vi "Composite User Interface Launcher.vi"   [LabVIEW 2020, in "2. Basic Panel Actors.lvlib"]
doc: "Launches the Composite UI Example\n----\nCopyright: MGI 2017\nAuthor: Derek Trepanier"
uses:
  2. Basic Panel Actors.lvlib
  Composite User Interface/Composite User Interface.lvclass
  C:/Program Files/National Instruments/LabVIEW 2020/vi.lib/MGI/Panel Manager/Panel Actor/Panel Actor/Panel Actor.lvclass
  <vilib>/MGI/Panel Manager/Panel/Window Position/Reference Position/Ref Display/Ref Display.lvclass
  C:/Program Files/National Instruments/LabVIEW 2020/vi.lib/MGI/Panel Manager/Panel/Window Position/Window Position.lvclass
  <vilib>/MGI/Panel Manager/Panel/Window Position/Reference Position/Ref Display/Ref Display.vi
  <vilib>/MGI/Panel Manager/Panel Actor/Panel Actor/Launch Root Panel Window.vi
  <vilib>/MGI/Panel Manager/Panel Actor/Panel Actor/Panel Actor.lvclass
  <vilib>/MGI/Panel Manager/Panel/Panel.lvlib
  C:/Program Files/National Instruments/LabVIEW 2020/vi.lib/MGI/Panel Manager/Panel/Window Position/Reference Position/Reference Position.lvclass
  C:/Program Files/National Instruments/LabVIEW 2020/vi.lib/MGI/Panel Manager/Panel/Window Position/Reference Position/Ref Display/Ref Display.lvclass
  C:/Program Files/National Instruments/LabVIEW 2020/vi.lib/MGI/Monitored Actor/Monitored Actor/Monitored Actor/Monitored Actor.lvclass
  C:/Program Files/National Instruments/LabVIEW 2020/vi.lib/ActorFramework/Actor/Actor.lvclass
  C:/Program Files/National Instruments/LabVIEW 2020/examples/MGI/Panel Manager/Basic Panel Actors/Composite User Interface/Composite User Interface/Composite User Interface.lvclass
panel:
  # "Run this VI to launch the Composite User Interface example."
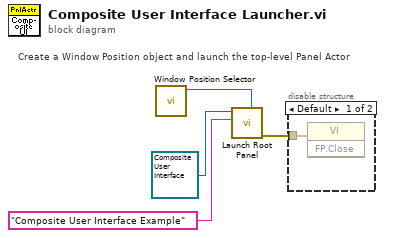
[diagram p0: block diagram]
diagram:
  # "Create a Window Position object and launch the top-level Panel Actor"
  n1 = call-poly <vilib>:"Window Position Selector.vi"() -> ("Ref Display out"=w1:refnum<class "Ref Display.lvclass">)  [unwired: 10 in, 1 out]
  n2 = call-poly <vilib>:"Launch Root Panel.vi"("Window Position (Maximize First Call)"=w1, "Title"="Composite User Interface Example", "Panel Actor in"=refnum<class "Composite User Interface.lvclass"> refnum ("2. Basic Panel Actors.lvlib:Composite User Interface.lvclass")) -> ("Error Out"=w2:errorcluster)  [unwired: 7 in, 1 out]
  n3 = disable-structure shown="Default" {
    disable-tunnel: w2 -> [w5 _]
    frame condition #0 {
      n4 = invoke class="VI" method="FP.Close"(error in=w5) -> ()  [unwired: 2 in, 3 out]
    }
    frame condition #1 (active) {
    }
  }
